vi "FTW-Subscriber-Construct.vi"(9 "Buffer Depth (1 element)":i32=1, 11 "error in":errorcluster) -> (4 "FTW-Subscription Out":refnum<class "FTW-Subscriber.lvclass">, 6 "Subscriber Registration":refnum<event-registration>, 15 "error out":errorcluster)   [LabVIEW 2015, in "FTW-Subscriber.lvclass"]
uses:
  FTW-Subscriber.lvclass
  Message/Base/FTW-Message.lvclass
  FTW-Subscriber.lvclass/FTW-Subscriber.ctl
  Message/Lossy/FTW-Message-Lossy.lvclass
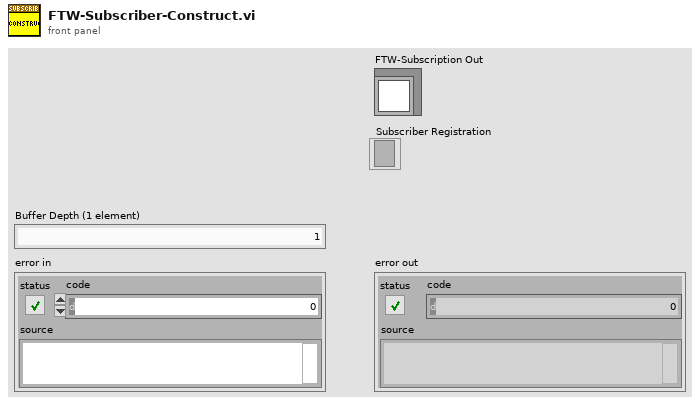
[diagram p1: front panel]
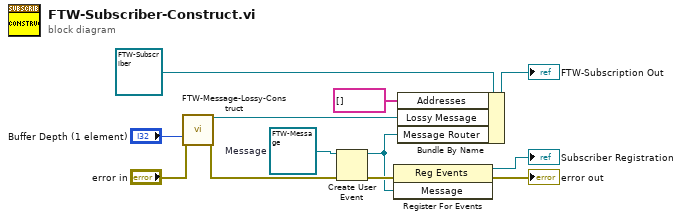
[diagram p0: block diagram]
diagram:
  w7 = refnum<class "FTW-Message.lvclass"> refnum  # Message
  n1 = call "FTW-Message-Lossy-Construct.vi"("max queue size (1)"="Buffer Depth (1 element)", "error in"="error in") -> ("FTW-Message-Lossy"=w1:refnum<class "FTW-Message-Lossy.lvclass">, "error out"=w2:errorcluster)  [unwired: 12 in]
  n2 = Create User Event(user event datatype=w7, error in=w2) -> (user event=w3:refnum<user-event>, error out=w6:errorcluster)
  n3 = register-events(error in=w6, w3) -> (reference out=→"Subscriber Registration":refnum<event-registration>, error out=→"error out":errorcluster)  [unwired: 1 in]
  n4 = Bundle By Name(cluster=refnum<class "FTW-Subscriber.lvclass"> refnum ("LVmsg_Router.lvclass"), "Addresses"=string[] [], "Lossy Message"=w1, "Message Router"=w3) -> (→"FTW-Subscription Out":refnum<class "FTW-Subscriber.lvclass">)
